vi "Init.vi"(8 "error in":errorcluster, 11 "PCAN Basic in":refnum<class "PCAN Basic Base Configure Strategy.lvclass">) -> (0 "error out":errorcluster, 3 "PCAN Basic out":refnum<class "PCAN Basic Base Configure Strategy.lvclass">)   [LabVIEW 2025, in "PCAN Basic Base Configure Strategy.lvclass"]
uses:
  PCAN Basic Base Configure Strategy.lvclass
  PCAN Basic Base Configure Strategy.lvclass/PCAN Basic Base Configure Strategy.ctl
  <instrlib>/Peter/PCAN Basic/TPCANHandle.ctl
  <instrlib>/Peter/PCAN Basic/PCAN Baud.ctl
  Source/Interfaces/IConfiguration/IConfiguration.lvclass
  <instrlib>/Peter/PCAN Basic/PCANBasic.lvlib
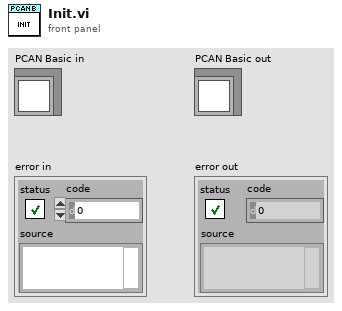
[diagram p1: front panel]
types:
  T1 = typedef "PCANBasic.lvlib/TPCANHandle.ctl" = u16
  T2 = typedef "PCANBasic.lvlib/PCAN Baud.ctl" = u16
  T3 = enum16{"PCAN_CHANNEL_UNAVAILABLE", "PCAN_CHANNEL_AVAILABLE", "PCAN_CHANNEL_OCCUPIED"}
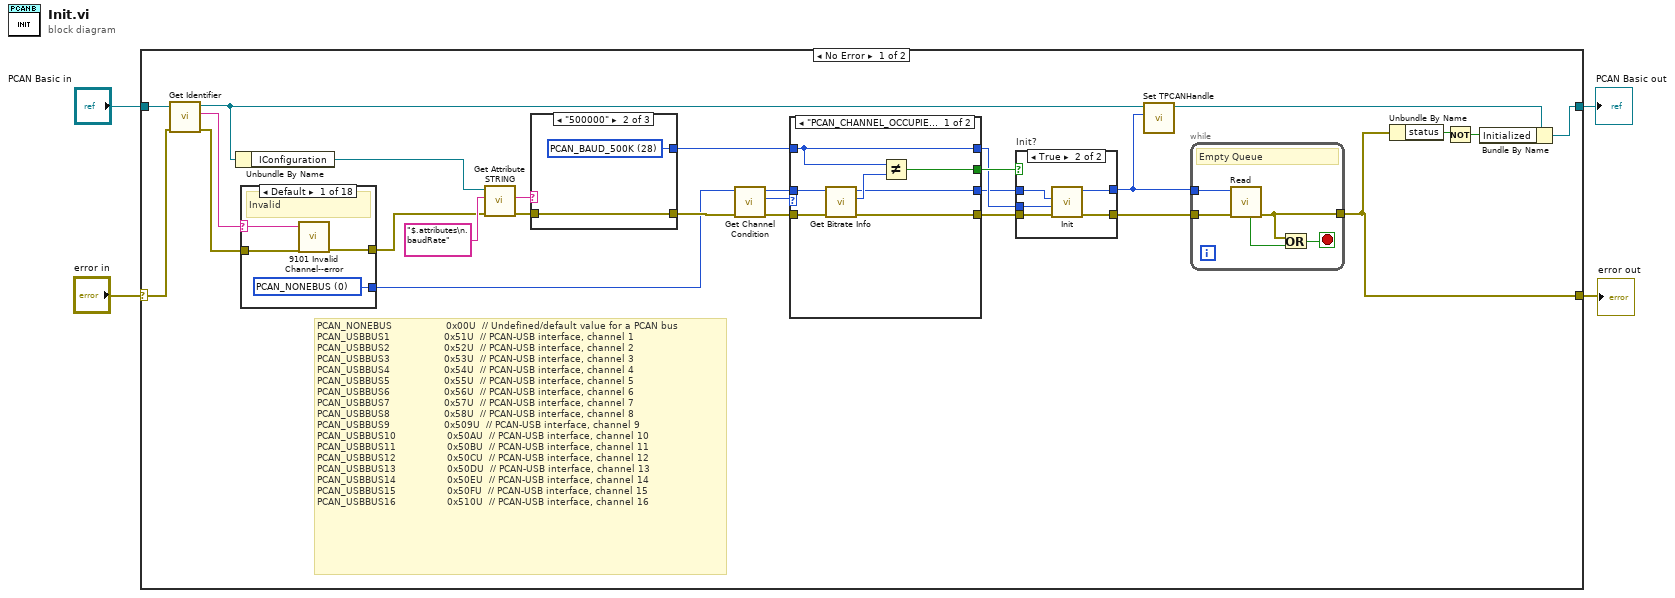
[diagram p0: block diagram]
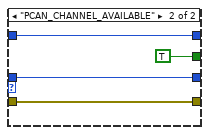
[diagram p2: hidden frame]
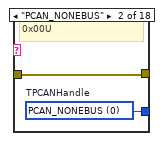
[diagram p3: hidden frame]
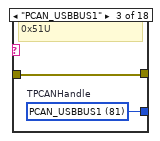
[diagram p4: hidden frame]
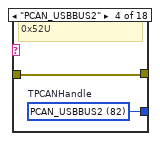
[diagram p5: hidden frame]
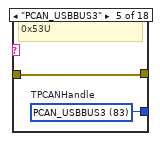
[diagram p6: hidden frame]
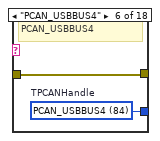
[diagram p7: hidden frame]
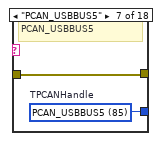
[diagram p8: hidden frame]
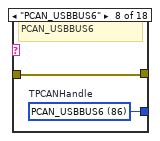
[diagram p9: hidden frame]
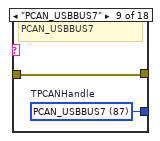
[diagram p10: hidden frame]
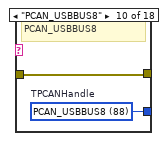
[diagram p11: hidden frame]
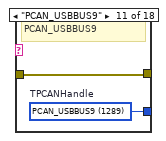
[diagram p12: hidden frame]
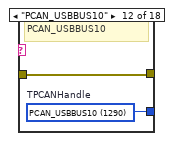
[diagram p13: hidden frame]
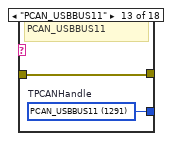
[diagram p14: hidden frame]
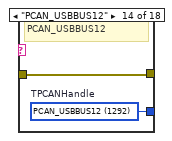
[diagram p15: hidden frame]
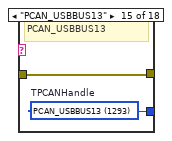
[diagram p16: hidden frame]
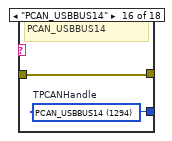
[diagram p17: hidden frame]
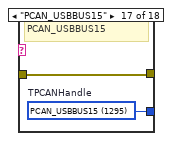
[diagram p18: hidden frame]
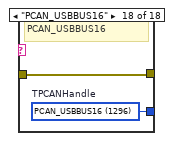
[diagram p19: hidden frame]
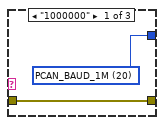
[diagram p20: hidden frame]
diagram:
  n1 = case shown="No Error" "error in" {
    selector: "error in" -> [w30 w100]
    tunnel: [w26 w100] -> w3
    tunnel: "PCAN Basic in" -> [w31 w101]
    tunnel: [w17 w101] -> w1
    frame No Error {
      # "PCAN_NONEBUS                  0x00U  // Undefined/default value for a PCAN bus\nPCAN_USBBUS1                  0x51U  // PCAN-USB interface, channel 1\nPCAN_USBBUS2                  0x52U  // PCAN-USB interface, channel 2\nPCAN_USBBUS3                  0x53U  // PCAN-USB interface, channel 3\nPCAN_USBBUS4                  0x54U  // PCAN-USB interface, channel 4\nPCAN_USBBUS5                  0x55U  // PCAN-USB interface, channel 5\nPCAN_USBBUS6                  0x56U  // PCAN-USB interface, channel 6\nPCAN_USBBUS7                  0x57U  // PCAN-USB interface, channel 7\nPCAN_USBBUS8                  0x58U  // PCAN-USB interface, channel 8\nPCAN_USBBUS9                  0x509U  // PCAN-USB interface, channel 9\nPCAN_USBBUS10                 0x50AU  // PCAN-USB interface, channel 10\nPCAN_USBBUS11                 0x50BU  // PCAN-USB interface, channel 11\nPCAN_USBBUS12                 0x50CU  // PCAN-USB interface, channel 12\nPCAN_USBBUS13                 0x50DU  // PCAN-USB interface, channel 13\nPCAN_USBBUS14                 0x50EU  // PCAN-USB interface, channel 14\nPCAN_USBBUS15                 0x50FU  // PCAN-USB interface, channel 15\nPCAN_USBBUS16                 0x510U  // PCAN-USB interface, channel 16"
      n2 = call-dynamic "Get Identifier.vi"("error in"=w30, "PCAN Basic in"=w31) -> ("error out"=w20:errorcluster, "Identifier"=w21:string, "PCAN Basic out"=w18:refnum<class "PCAN Basic Base Configure Strategy.lvclass">)  [unwired: 7 in]
      n3 = Unbundle By Name(w18) -> ("IConfiguration"=w25:refnum<class "IConfiguration.lvclass">)
      n4 = case shown="Default" w21 {
        selector: w21 -> [w45 _ _ _ _ _ _ _ _ _ _ _ _ _ _ _ _ _]
        tunnel: w20 -> [w46 w48 w50 w52 w54 w56 w58 w60 w62 w64 w66 w68 w70 w72 w74 w76 w78 w80]
        tunnel: [w44 w48 w50 w52 w54 w56 w58 w60 w62 w64 w66 w68 w70 w72 w74 w76 w78 w80] -> w19
        tunnel: [w43 w47 w49 w51 w53 w55 w57 w59 w61 w63 w65 w67 w69 w71 w73 w75 w77 w79] -> w9
        frame Default {
          w43 = T1 0 items=["PCAN_NONEBUS"=0, "PCAN_USBBUS1"=81, "PCAN_USBBUS2"=82, "PCAN_USBBUS3"=83, "PCAN_USBBUS4"=84, "PCAN_USBBUS5"=85, "PCAN_USBBUS6"=86, "PCAN_USBBUS7"=87, "PCAN_USBBUS8"=88, "PCAN_USBBUS9"=1289, "PCAN_USBBUS10"=1290, "PCAN_USBBUS11"=1291, "PCAN_USBBUS12"=1292, "PCAN_USBBUS13"=1293, "PCAN_USBBUS14"=1294, "PCAN_USBBUS15"=1295, "PCAN_USBBUS16"=1296] ("TPCANHandle")
          # "Invalid"
          n5 = call "9101 Invalid Channel--error.vi"("error in"=w46, "Argument"=w45) -> ("error out"=w44:errorcluster)  [unwired: 8 in, 1 out]
        }
        frame "PCAN_NONEBUS" {
          w47 = T1 0 items=["PCAN_NONEBUS"=0, "PCAN_USBBUS1"=81, "PCAN_USBBUS2"=82, "PCAN_USBBUS3"=83, "PCAN_USBBUS4"=84, "PCAN_USBBUS5"=85, "PCAN_USBBUS6"=86, "PCAN_USBBUS7"=87, "PCAN_USBBUS8"=88, "PCAN_USBBUS9"=1289, "PCAN_USBBUS10"=1290, "PCAN_USBBUS11"=1291, "PCAN_USBBUS12"=1292, "PCAN_USBBUS13"=1293, "PCAN_USBBUS14"=1294, "PCAN_USBBUS15"=1295, "PCAN_USBBUS16"=1296]  # TPCANHandle
          # "0x00U"
        }
        frame "PCAN_USBBUS1" {
          w49 = T1 81 items=["PCAN_NONEBUS"=0, "PCAN_USBBUS1"=81, "PCAN_USBBUS2"=82, "PCAN_USBBUS3"=83, "PCAN_USBBUS4"=84, "PCAN_USBBUS5"=85, "PCAN_USBBUS6"=86, "PCAN_USBBUS7"=87, "PCAN_USBBUS8"=88, "PCAN_USBBUS9"=1289, "PCAN_USBBUS10"=1290, "PCAN_USBBUS11"=1291, "PCAN_USBBUS12"=1292, "PCAN_USBBUS13"=1293, "PCAN_USBBUS14"=1294, "PCAN_USBBUS15"=1295, "PCAN_USBBUS16"=1296]  # TPCANHandle
          # "0x51U"
        }
        frame "PCAN_USBBUS2" {
          w51 = T1 82 items=["PCAN_NONEBUS"=0, "PCAN_USBBUS1"=81, "PCAN_USBBUS2"=82, "PCAN_USBBUS3"=83, "PCAN_USBBUS4"=84, "PCAN_USBBUS5"=85, "PCAN_USBBUS6"=86, "PCAN_USBBUS7"=87, "PCAN_USBBUS8"=88, "PCAN_USBBUS9"=1289, "PCAN_USBBUS10"=1290, "PCAN_USBBUS11"=1291, "PCAN_USBBUS12"=1292, "PCAN_USBBUS13"=1293, "PCAN_USBBUS14"=1294, "PCAN_USBBUS15"=1295, "PCAN_USBBUS16"=1296]  # TPCANHandle
          # "0x52U"
        }
        frame "PCAN_USBBUS3" {
          w53 = T1 83 items=["PCAN_NONEBUS"=0, "PCAN_USBBUS1"=81, "PCAN_USBBUS2"=82, "PCAN_USBBUS3"=83, "PCAN_USBBUS4"=84, "PCAN_USBBUS5"=85, "PCAN_USBBUS6"=86, "PCAN_USBBUS7"=87, "PCAN_USBBUS8"=88, "PCAN_USBBUS9"=1289, "PCAN_USBBUS10"=1290, "PCAN_USBBUS11"=1291, "PCAN_USBBUS12"=1292, "PCAN_USBBUS13"=1293, "PCAN_USBBUS14"=1294, "PCAN_USBBUS15"=1295, "PCAN_USBBUS16"=1296]  # TPCANHandle
          # "0x53U"
        }
        frame "PCAN_USBBUS4" {
          w55 = T1 84 items=["PCAN_NONEBUS"=0, "PCAN_USBBUS1"=81, "PCAN_USBBUS2"=82, "PCAN_USBBUS3"=83, "PCAN_USBBUS4"=84, "PCAN_USBBUS5"=85, "PCAN_USBBUS6"=86, "PCAN_USBBUS7"=87, "PCAN_USBBUS8"=88, "PCAN_USBBUS9"=1289, "PCAN_USBBUS10"=1290, "PCAN_USBBUS11"=1291, "PCAN_USBBUS12"=1292, "PCAN_USBBUS13"=1293, "PCAN_USBBUS14"=1294, "PCAN_USBBUS15"=1295, "PCAN_USBBUS16"=1296]  # TPCANHandle
          # "PCAN_USBBUS4"
        }
        frame "PCAN_USBBUS5" {
          w57 = T1 85 items=["PCAN_NONEBUS"=0, "PCAN_USBBUS1"=81, "PCAN_USBBUS2"=82, "PCAN_USBBUS3"=83, "PCAN_USBBUS4"=84, "PCAN_USBBUS5"=85, "PCAN_USBBUS6"=86, "PCAN_USBBUS7"=87, "PCAN_USBBUS8"=88, "PCAN_USBBUS9"=1289, "PCAN_USBBUS10"=1290, "PCAN_USBBUS11"=1291, "PCAN_USBBUS12"=1292, "PCAN_USBBUS13"=1293, "PCAN_USBBUS14"=1294, "PCAN_USBBUS15"=1295, "PCAN_USBBUS16"=1296]  # TPCANHandle
          # "PCAN_USBBUS5"
        }
        frame "PCAN_USBBUS6" {
          w59 = T1 86 items=["PCAN_NONEBUS"=0, "PCAN_USBBUS1"=81, "PCAN_USBBUS2"=82, "PCAN_USBBUS3"=83, "PCAN_USBBUS4"=84, "PCAN_USBBUS5"=85, "PCAN_USBBUS6"=86, "PCAN_USBBUS7"=87, "PCAN_USBBUS8"=88, "PCAN_USBBUS9"=1289, "PCAN_USBBUS10"=1290, "PCAN_USBBUS11"=1291, "PCAN_USBBUS12"=1292, "PCAN_USBBUS13"=1293, "PCAN_USBBUS14"=1294, "PCAN_USBBUS15"=1295, "PCAN_USBBUS16"=1296]  # TPCANHandle
          # "PCAN_USBBUS6"
        }
        frame "PCAN_USBBUS7" {
          w61 = T1 87 items=["PCAN_NONEBUS"=0, "PCAN_USBBUS1"=81, "PCAN_USBBUS2"=82, "PCAN_USBBUS3"=83, "PCAN_USBBUS4"=84, "PCAN_USBBUS5"=85, "PCAN_USBBUS6"=86, "PCAN_USBBUS7"=87, "PCAN_USBBUS8"=88, "PCAN_USBBUS9"=1289, "PCAN_USBBUS10"=1290, "PCAN_USBBUS11"=1291, "PCAN_USBBUS12"=1292, "PCAN_USBBUS13"=1293, "PCAN_USBBUS14"=1294, "PCAN_USBBUS15"=1295, "PCAN_USBBUS16"=1296]  # TPCANHandle
          # "PCAN_USBBUS7"
        }
        frame "PCAN_USBBUS8" {
          w63 = T1 88 items=["PCAN_NONEBUS"=0, "PCAN_USBBUS1"=81, "PCAN_USBBUS2"=82, "PCAN_USBBUS3"=83, "PCAN_USBBUS4"=84, "PCAN_USBBUS5"=85, "PCAN_USBBUS6"=86, "PCAN_USBBUS7"=87, "PCAN_USBBUS8"=88, "PCAN_USBBUS9"=1289, "PCAN_USBBUS10"=1290, "PCAN_USBBUS11"=1291, "PCAN_USBBUS12"=1292, "PCAN_USBBUS13"=1293, "PCAN_USBBUS14"=1294, "PCAN_USBBUS15"=1295, "PCAN_USBBUS16"=1296]  # TPCANHandle
          # "PCAN_USBBUS8"
        }
        frame "PCAN_USBBUS9" {
          w65 = T1 1289 items=["PCAN_NONEBUS"=0, "PCAN_USBBUS1"=81, "PCAN_USBBUS2"=82, "PCAN_USBBUS3"=83, "PCAN_USBBUS4"=84, "PCAN_USBBUS5"=85, "PCAN_USBBUS6"=86, "PCAN_USBBUS7"=87, "PCAN_USBBUS8"=88, "PCAN_USBBUS9"=1289, "PCAN_USBBUS10"=1290, "PCAN_USBBUS11"=1291, "PCAN_USBBUS12"=1292, "PCAN_USBBUS13"=1293, "PCAN_USBBUS14"=1294, "PCAN_USBBUS15"=1295, "PCAN_USBBUS16"=1296]  # TPCANHandle
          # "PCAN_USBBUS9"
        }
        frame "PCAN_USBBUS10" {
          w67 = T1 1290 items=["PCAN_NONEBUS"=0, "PCAN_USBBUS1"=81, "PCAN_USBBUS2"=82, "PCAN_USBBUS3"=83, "PCAN_USBBUS4"=84, "PCAN_USBBUS5"=85, "PCAN_USBBUS6"=86, "PCAN_USBBUS7"=87, "PCAN_USBBUS8"=88, "PCAN_USBBUS9"=1289, "PCAN_USBBUS10"=1290, "PCAN_USBBUS11"=1291, "PCAN_USBBUS12"=1292, "PCAN_USBBUS13"=1293, "PCAN_USBBUS14"=1294, "PCAN_USBBUS15"=1295, "PCAN_USBBUS16"=1296]  # TPCANHandle
          # "PCAN_USBBUS10"
        }
        frame "PCAN_USBBUS11" {
          w69 = T1 1291 items=["PCAN_NONEBUS"=0, "PCAN_USBBUS1"=81, "PCAN_USBBUS2"=82, "PCAN_USBBUS3"=83, "PCAN_USBBUS4"=84, "PCAN_USBBUS5"=85, "PCAN_USBBUS6"=86, "PCAN_USBBUS7"=87, "PCAN_USBBUS8"=88, "PCAN_USBBUS9"=1289, "PCAN_USBBUS10"=1290, "PCAN_USBBUS11"=1291, "PCAN_USBBUS12"=1292, "PCAN_USBBUS13"=1293, "PCAN_USBBUS14"=1294, "PCAN_USBBUS15"=1295, "PCAN_USBBUS16"=1296]  # TPCANHandle
          # "PCAN_USBBUS11"
        }
        frame "PCAN_USBBUS12" {
          w71 = T1 1292 items=["PCAN_NONEBUS"=0, "PCAN_USBBUS1"=81, "PCAN_USBBUS2"=82, "PCAN_USBBUS3"=83, "PCAN_USBBUS4"=84, "PCAN_USBBUS5"=85, "PCAN_USBBUS6"=86, "PCAN_USBBUS7"=87, "PCAN_USBBUS8"=88, "PCAN_USBBUS9"=1289, "PCAN_USBBUS10"=1290, "PCAN_USBBUS11"=1291, "PCAN_USBBUS12"=1292, "PCAN_USBBUS13"=1293, "PCAN_USBBUS14"=1294, "PCAN_USBBUS15"=1295, "PCAN_USBBUS16"=1296]  # TPCANHandle
          # "PCAN_USBBUS12"
        }
        frame "PCAN_USBBUS13" {
          w73 = T1 1293 items=["PCAN_NONEBUS"=0, "PCAN_USBBUS1"=81, "PCAN_USBBUS2"=82, "PCAN_USBBUS3"=83, "PCAN_USBBUS4"=84, "PCAN_USBBUS5"=85, "PCAN_USBBUS6"=86, "PCAN_USBBUS7"=87, "PCAN_USBBUS8"=88, "PCAN_USBBUS9"=1289, "PCAN_USBBUS10"=1290, "PCAN_USBBUS11"=1291, "PCAN_USBBUS12"=1292, "PCAN_USBBUS13"=1293, "PCAN_USBBUS14"=1294, "PCAN_USBBUS15"=1295, "PCAN_USBBUS16"=1296]  # TPCANHandle
          # "PCAN_USBBUS13"
        }
        frame "PCAN_USBBUS14" {
          w75 = T1 1294 items=["PCAN_NONEBUS"=0, "PCAN_USBBUS1"=81, "PCAN_USBBUS2"=82, "PCAN_USBBUS3"=83, "PCAN_USBBUS4"=84, "PCAN_USBBUS5"=85, "PCAN_USBBUS6"=86, "PCAN_USBBUS7"=87, "PCAN_USBBUS8"=88, "PCAN_USBBUS9"=1289, "PCAN_USBBUS10"=1290, "PCAN_USBBUS11"=1291, "PCAN_USBBUS12"=1292, "PCAN_USBBUS13"=1293, "PCAN_USBBUS14"=1294, "PCAN_USBBUS15"=1295, "PCAN_USBBUS16"=1296]  # TPCANHandle
          # "PCAN_USBBUS14"
        }
        frame "PCAN_USBBUS15" {
          w77 = T1 1295 items=["PCAN_NONEBUS"=0, "PCAN_USBBUS1"=81, "PCAN_USBBUS2"=82, "PCAN_USBBUS3"=83, "PCAN_USBBUS4"=84, "PCAN_USBBUS5"=85, "PCAN_USBBUS6"=86, "PCAN_USBBUS7"=87, "PCAN_USBBUS8"=88, "PCAN_USBBUS9"=1289, "PCAN_USBBUS10"=1290, "PCAN_USBBUS11"=1291, "PCAN_USBBUS12"=1292, "PCAN_USBBUS13"=1293, "PCAN_USBBUS14"=1294, "PCAN_USBBUS15"=1295, "PCAN_USBBUS16"=1296]  # TPCANHandle
          # "PCAN_USBBUS15"
        }
        frame "PCAN_USBBUS16" {
          w79 = T1 1296 items=["PCAN_NONEBUS"=0, "PCAN_USBBUS1"=81, "PCAN_USBBUS2"=82, "PCAN_USBBUS3"=83, "PCAN_USBBUS4"=84, "PCAN_USBBUS5"=85, "PCAN_USBBUS6"=86, "PCAN_USBBUS7"=87, "PCAN_USBBUS8"=88, "PCAN_USBBUS9"=1289, "PCAN_USBBUS10"=1290, "PCAN_USBBUS11"=1291, "PCAN_USBBUS12"=1292, "PCAN_USBBUS13"=1293, "PCAN_USBBUS14"=1294, "PCAN_USBBUS15"=1295, "PCAN_USBBUS16"=1296]  # TPCANHandle
          # "PCAN_USBBUS16"
        }
      }
      n6 = call-dynamic "Get Attribute STRING.vi"("error in"=w19, "Attribute"="$.attributes\n.baudRate", "IConfiguration in"=w25) -> ("error out"=w23:errorcluster, "Value"=w22:string)  [unwired: 6 in, 1 out]
      n7 = case shown="\"500000\"" w22 {
        selector: w22 -> [_ _ w85]
        tunnel: [w82 w84 _] -> w11
        tunnel: w23 -> [w81 w83 w87]
        tunnel: [w81 w83 w86] -> w15
        frame "1000000" {
          w82 = T2 20 items=["PCAN_BAUD_1M"=20, "PCAN_BAUD_800K"=22, "PCAN_BAUD_500K"=28, "PCAN_BAUD_250K"=284, "PCAN_BAUD_125K"=796, "PCAN_BAUD_100K"=17199, "PCAN_BAUD_95K"=49998, "PCAN_BAUD_83K"=34091, "PCAN_BAUD_50K"=18223, "PCAN_BAUD_47K"=5140, "PCAN_BAUD_33K"=35631, "PCAN_BAUD_20K"=21295, "PCAN_BAUD_10K"=26415, "PCAN_BAUD_5K"=32639] ("Baudrate")
        }
        frame "500000" {
          w84 = T2 28 items=["PCAN_BAUD_1M"=20, "PCAN_BAUD_800K"=22, "PCAN_BAUD_500K"=28, "PCAN_BAUD_250K"=284, "PCAN_BAUD_125K"=796, "PCAN_BAUD_100K"=17199, "PCAN_BAUD_95K"=49998, "PCAN_BAUD_83K"=34091, "PCAN_BAUD_50K"=18223, "PCAN_BAUD_47K"=5140, "PCAN_BAUD_33K"=35631, "PCAN_BAUD_20K"=21295, "PCAN_BAUD_10K"=26415, "PCAN_BAUD_5K"=32639] ("Baudrate")
        }
        frame Default {
          n8 = call "9100 Baudrate not implemented--error.vi"("error in"=w87, "Argument"=w85) -> ("error out"=w86:errorcluster)  [unwired: 9 in]
        }
      }
      n9 = call <instrlib>:"Get Channel Condition.vi"("error in"=w15, "TPCANHandle in"=w9) -> ("error out"=w14:errorcluster, "Channel Condition"=w10:T3, "TPCANHandle out"=w13:T1)  [unwired: 6 in, 1 out]
      n10 = case shown="\"PCAN_CHANNEL_OCCUPIED\", Default" w10 {
        tunnel: w14 -> [w38 w42]
        tunnel: w13 -> [w36 w39]
        tunnel: [w37 w42] -> w12
        tunnel: w11 -> [w33 w40]
        tunnel: [w34 TRUE] -> w8
        tunnel: [w33 w40] -> w7
        tunnel: [w32 w39] -> w6
        frame "PCAN_CHANNEL_OCCUPIED", Default {
          n11 = call <instrlib>:"Get Bitrate Info.vi"("error in"=w38, "TPCANHandle in"=w36) -> ("error out"=w37:errorcluster, "Baudrate"=w35:T2, "TPCANHandle out"=w32:T1)  [unwired: 6 in, 1 out]
          n12 = Not Equal?(x=w33, y=w35) -> (x != y?=w34:bool)
        }
        frame "PCAN_CHANNEL_AVAILABLE" {
        }
      }
      n13 = case "Init?" shown="True" w8 {
        tunnel: [w89 w94] -> w29
        tunnel: [w88 w93] -> w5
        tunnel: w12 -> [w89 w92]
        tunnel: w7 -> [_ w91]
        tunnel: w6 -> [w88 w90]
        frame False {
        }
        frame True {
          n14 = call <instrlib>:"Init.vi"("error in"=w92, "Baudrate"=w91, "Channel"=w90) -> ("error out"=w94:errorcluster, "TPCANHandle out"=w93:T1)  [unwired: 6 in, 1 out]
        }
      }
      n15 = call "Set TPCANHandle.vi"("TPCANHandle"=w5, "PCAN Basic Base Configure Strategy in"=w18) -> ("PCAN Basic Base Configure Strategy out"=w16:refnum<class "PCAN Basic Base Configure Strategy.lvclass">)  [unwired: 9 in]
      n16 = while {
        tunnel: w29 -> [w99]
        tunnel: w5 -> [w98]
        tunnel: [w96] -> w26
        stop <- w97 stop-if-true
        # "Empty Queue"
        n17 = call <instrlib>:"Read.vi"("error in"=w99, "TPCANHandle in"=w98) -> ("error out"=w96:errorcluster, "Receive Queue empty"=w95:bool)  [unwired: 4 in, 4 out]
        n18 = Or(x=w96, y=w95) -> (x .or. y?=w97:bool)
      }
      n19 = Unbundle By Name(w26) -> ("status"=w28:bool)
      n20 = Not(x=w28) -> (.not. x?=w27:bool)
      n21 = Bundle By Name(cluster=w16, "Initialized"=w27) -> (w17:refnum<class "PCAN Basic Base Configure Strategy.lvclass">)
    }
    frame Error {
    }
  }
  "error out" <- w3
  "PCAN Basic out" <- w1
